vi "ST Speed.vi"(4 "error in (error out)":errorcluster, 5 "New Speed":string, 6 "Action":string(combo)="OFF", 7 "VISA resource name in":refnum<visa-resource-name>) -> (0 "error out":errorcluster, 1 "Motor Speed":string, 2 "Complete":bool, 3 "VISA resource name out":refnum<visa-resource-name>)   [LabVIEW 2009]
doc: "This VI either sets or gets the motor speed in steps. The input and output are strings\nValues are:\n1000 slow\n10000 medium\n30000 high\nValues must be greater than 16X the acceleration value"
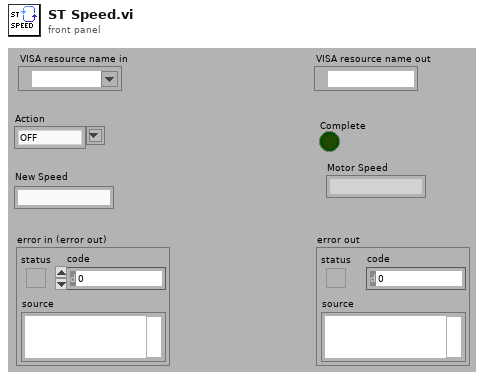
[diagram p1: front panel]
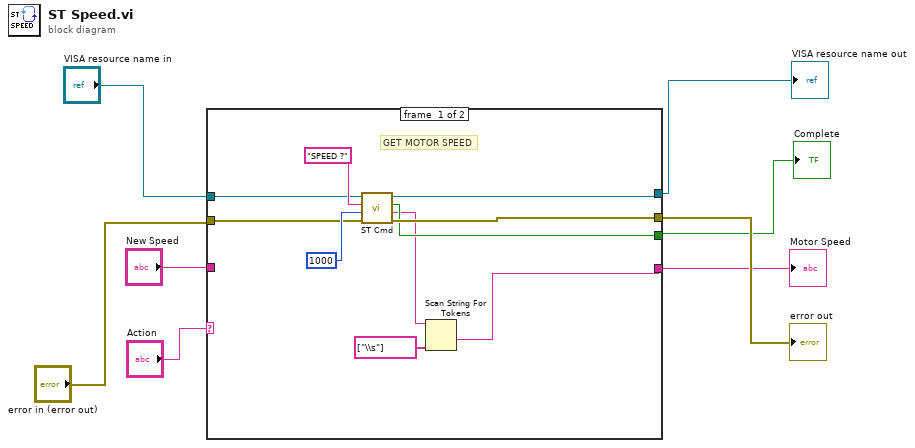
[diagram p0: block diagram]
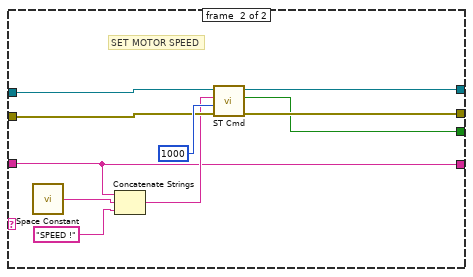
[diagram p2: hidden frame]
diagram:
  n1 = case shown="\"SET\"" "Action" {
    tunnel: [w14 w28] -> w8
    tunnel: [w13 w27] -> w7
    tunnel: [w12 w26] -> w3
    tunnel: "VISA resource name in" -> [w16 w24]
    tunnel: "error in (error out)" -> [w15 w23]
    tunnel: "New Speed" -> [_ w19]
    tunnel: [w9 w19] -> w1
    frame #0 {
      # "GET MOTOR SPEED"
      n2 = call "ST Cmd.vi"("error in (no error)"=w15, "Time Out"=1000, "Command String"="SPEED ?", "VISA resource name"=w16) -> ("error out"=w13:errorcluster, "String Received"=w10:string, "Ready and OK"=w12:bool, "VISA resource name out"=w14:refnum<visa-resource-name>)  [unwired: 1 out]
      n3 = Scan String For Tokens(6:string[] ["\\s"] ("delimiters (\\s,\\t,\\r,\\n)"), 9:w10) -> (1:w9:string)  [unwired: 4 in, 3 out]
    }
    frame #1 {
      # "SET MOTOR SPEED"
      n4 = call <vilib>:"Space Constant.vi"() -> ("String"=w22:string)
      n5 = Concatenate Strings(w19, w22, "SPEED !" ("Command String")) -> (w20:string)
      n6 = call "ST Cmd.vi"("error in (no error)"=w23, "Time Out"=1000, "Command String"=w20, "VISA resource name"=w24) -> ("error out"=w27:errorcluster, "Ready and OK"=w26:bool, "VISA resource name out"=w28:refnum<visa-resource-name>)  [unwired: 2 out]
    }
  }
  "VISA resource name out" <- w8
  "error out" <- w7
  "Complete" <- w3
  "Motor Speed" <- w1
